vi "Log Autobalance Algorithm State.vi"(9 "Records In":string, 10 "Autobalance State":T1[](array[typedef])) -> (1 "Records Out":string)   [LabVIEW 2009]
uses:
  lib/Autobalance/Autobalance Status Data.ctl
  lib/Apps/Yes No Button.ctl
  lib/Autobalance/Autobalance Stage.ctl
  lib/Autobalance/Autobalance Data Point.ctl
panel:
  # "Cmd"
  # "Servo"
  # "Cmd"
  # "Servo"
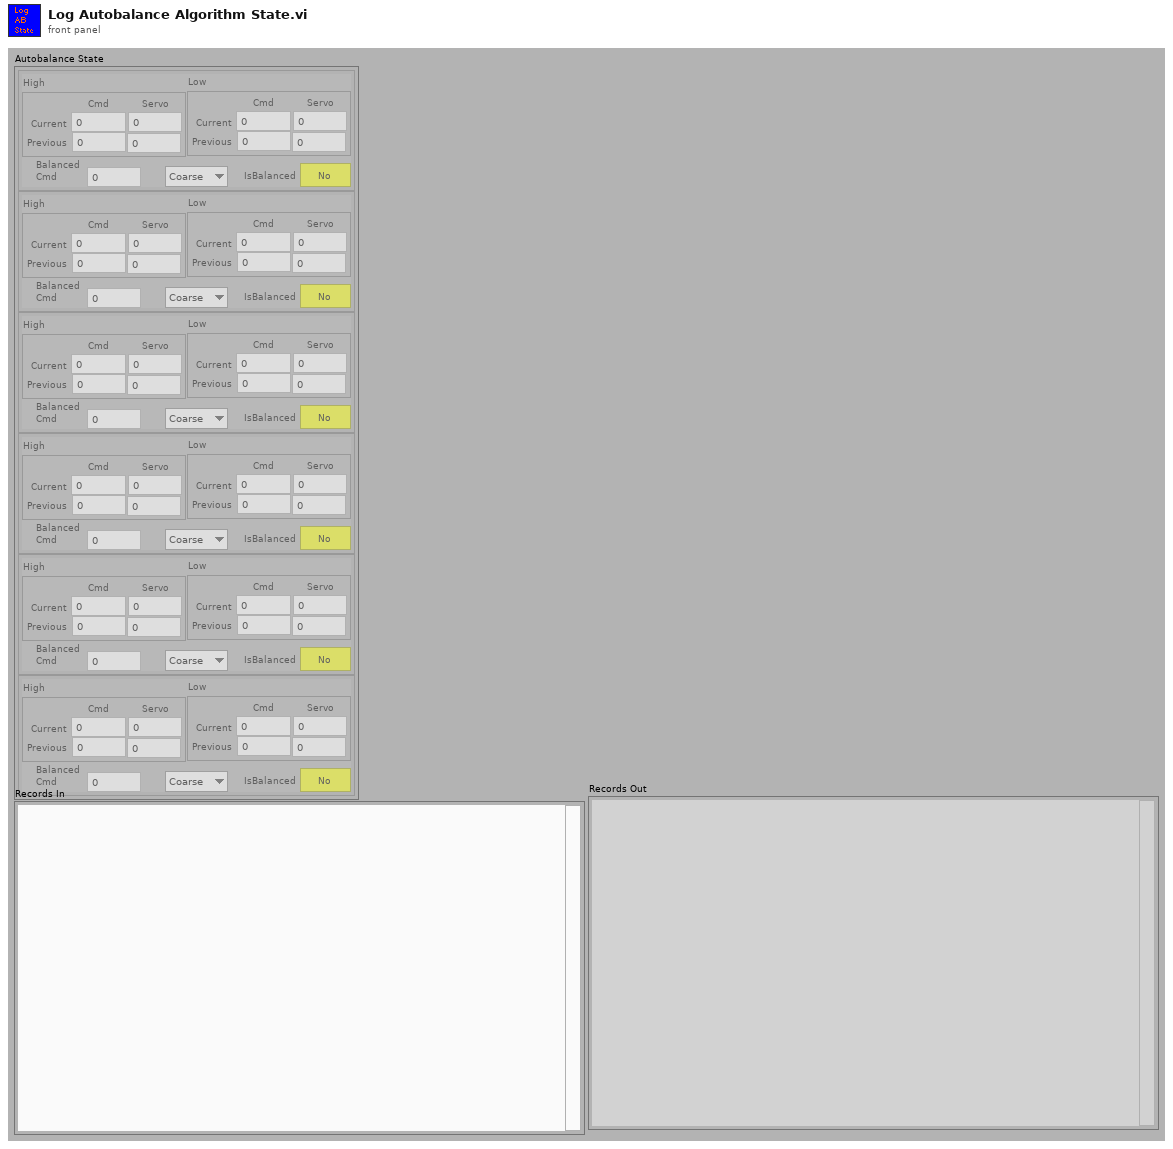
[diagram p1: front panel]
types:
  T1 = typedef "Autobalance Status Data.ctl" = cluster{"IsBalanced":T2, "Autobalance Stage":T3, "High":T4, "Low":T4, "Balanced \nCmd":dbl}
  T2 = typedef "Yes No Button.ctl" = bool
  T3 = typedef "Autobalance Stage.ctl" = enum16{"Coarse", "Fine", "Backing Up", "Done"}
  T4 = typedef "Autobalance Data Point.ctl" = cluster{"cCmd":dbl, "cServo":dbl, "pCmd":dbl, "pServo":dbl}
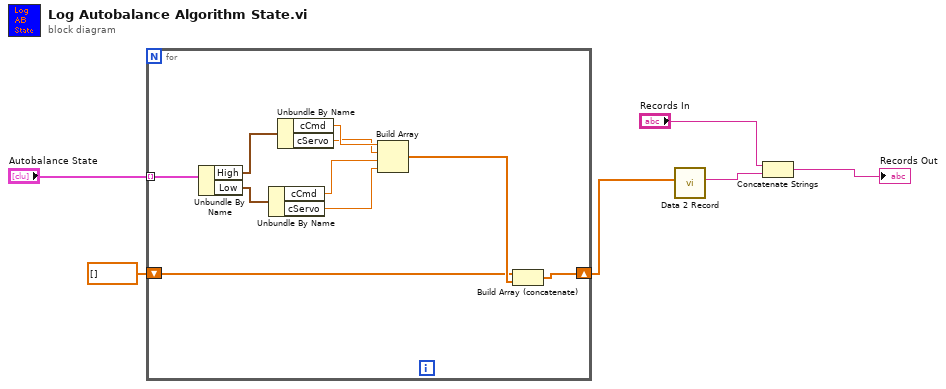
[diagram p0: block diagram]
diagram:
  n1 = for {
    tunnel: "Autobalance State" -> [w16] mode=indexing
    shift-right: [w8] -> w5
    shift-left: dbl[] [] -> [w7]
    n2 = Unbundle By Name(w16) -> ("High"=w15:T4, "Low"=w14:T4)
    n3 = Unbundle By Name(w14) -> ("cCmd"=w11:dbl, "cServo"=w10:dbl)
    n4 = Unbundle By Name(w15) -> ("cCmd"=w13:dbl, "cServo"=w12:dbl)
    n5 = Build Array(w13, w12, w11, w10) -> (w9:dbl[])
    n6 = Build Array (concatenate)(w7, w9) -> (w8:dbl[])
  }
  n7 = call "Data 2 Record.vi"("Data"=w5) -> ("Records"=w3:string)  [unwired: 1 in, 9 out]
  n8 = Concatenate Strings("Records In", w3) -> (→"Records Out":string)
